vi "Start Simulation.vi"() -> ()   [LabVIEW 2018]
doc: "Imports MAX Configuration from specified location."
uses:
  <vilib>/Utility/error.llb/DialogType.ctl
  <vilib>/nisyscfg/Close (System).vi
  <vilib>/nisyscfg/nisyscfg.lvlib
panel:
  in  "User Name":string
  in  "Password":string
  in  "Target (localhost)":refnum<k21>="localhost"
  out "Detailed Result":string
  in  "Import Mode":u32(ring)=1048576 items=["merge"=0, "replace all"=1048576, "preserve existing"=2097152]
  # "Overview: Imports MAX Configuration from a specified location.\nRequirements: NI System Configuration, NI MAX\nInstructions:\n1. Select Target. Enter User Name and Password if necessary.\n2. Specify the location of the configuration file in File Path. \n3. Run the VI."
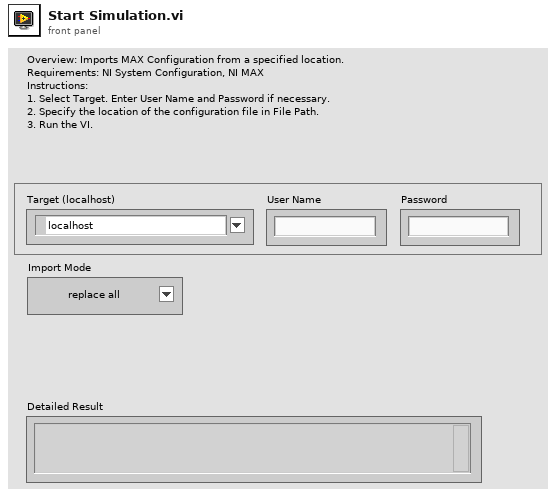
[diagram p1: front panel]
types:
  T1 = typedef "DialogType.ctl" = u16
  T2 = enum32{"invalid app kind", "Development System", "Run Time System", "Student Edition", "Embedded LabVIEW", "Evaluation", "Custom"}
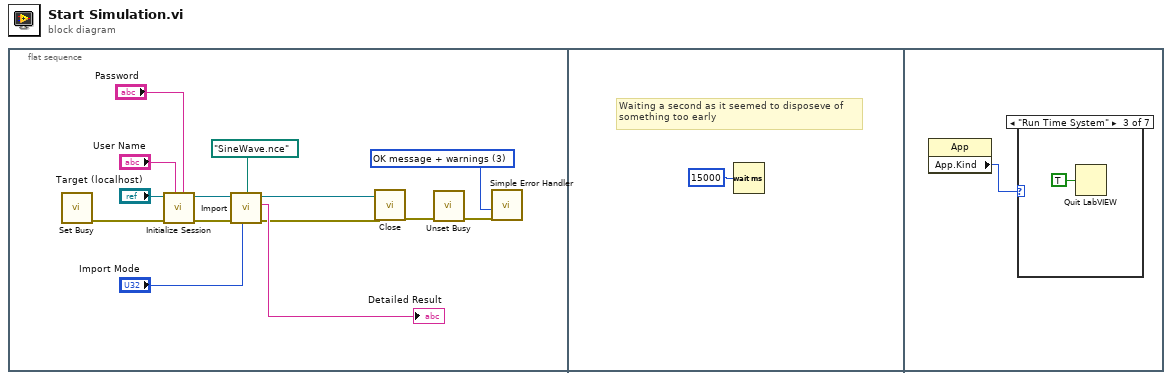
[diagram p0: block diagram]
diagram:
  n1 = flat-sequence {
    frame #0 {
      w9 = T1 3 items=["no dialog", "OK message", "continue or stop message", "OK message + warnings", "continue/stop + warnings"] ("type of dialog (OK msg:1)")
      n2 = call <vilib>:"Set Busy.vi"() -> ("error out"=w6:errorcluster)  [unwired: 10 in, 1 out]
      n3 = call <vilib>:"Initialize Session.vi"("Password"="Password", "User Name"="User Name", "error in (no error)"=w6, "Target (localhost)"="Target (localhost)") -> ("error out"=w5:errorcluster, "Session out"=w14:refnum<k21>)  [unwired: 6 in]
      n4 = call <vilib>:"Import.vi"("Import Mode"="Import Mode", "error in (no error)"=w5, "Source File"=path "SineWave.nce", "Session in"=w14) -> ("error out"=w3:errorcluster, "Detailed Result"=→"Detailed Result":string, "Session out"=w4:refnum<k21>)  [unwired: 5 in]
      n5 = call-poly <vilib>:"Close.vi"("error in (no error)"=w3, "Session in"=w4) -> ("error out"=w12:errorcluster)  [unwired: 9 in]
      n6 = call <vilib>:"Unset Busy.vi"("error in (no error)"=w12) -> ("error out"=w11:errorcluster)  [unwired: 10 in]
      n7 = call <vilib>:"Simple Error Handler.vi"("type of dialog (OK msg:1)"=w9, "error in (no error)"=w11) -> ()  [unwired: 3 in, 5 out]
    }
    frame #1 {
      # "Waiting a second as it seemed to disposeve of\nsomething too early"
      n8 = Wait (ms)(milliseconds to wait=u32 15000 ("millisecond multiple")) -> ()  [unwired: 1 out]
    }
    frame #2 {
      n9 = property class="App"() -> ("App.Kind"=w16:T2)  [unwired: 2 in, 2 out]
      n10 = case shown="\"Run Time System\"" w16 {
        frame "invalid app kind", Default {
        }
        frame "Development System" {
        }
        frame "Run Time System" {
          n11 = Quit LabVIEW(quit? (T)=TRUE) -> ()
        }
        frame "Student Edition" {
        }
        frame "Embedded LabVIEW" {
        }
        frame "Evaluation" {
        }
        frame "Custom" {
        }
      }
    }
  }
